vi "Camera Begin.vi"() -> ()   [LabVIEW 2013]
uses:
  <vilib>/Rock Robotics/WPI/Camera/WPI_CameraWhite Balance Values.ctl
  <vilib>/Rock Robotics/WPI/Camera/WPI_CameraFrameRate.ctl
  <vilib>/Rock Robotics/WPI/Camera/WPI_CameraExposure Values.ctl
  <vilib>/Rock Robotics/WPI/Camera/WPI_CameraImageSize.ctl
  <vilib>/Rock Robotics/SystemInterfaces/Typedef/FPGA_TypedefDigitalModule.ctl
  <vilib>/Rock Robotics/SystemInterfaces/DIO/FPGA_DIOPWMChannel.ctl
panel:
  in  "Camera 2":T5={"Camera Address"="192.168.0.90", "Compression"=0, "White Balance"=enum."Auto", "Frame Rate (fps)"=30, "Exposure"=enum."Auto", "Image Size"=enum."320x240", "Brightness"=50, "refnum name"="My Camera RefNum"} {"Brightness" min=0 max=100; "Frame Rate (fps)" min=1 max=30; "Compression" min=0 max=100}
  in  "Camera 1":T5={"Camera Address"="192.168.0.90", "Compression"=0, "White Balance"=enum."Auto", "Frame Rate (fps)"=30, "Exposure"=enum."Auto", "Image Size"=enum."320x240", "Brightness"=50, "refnum name"="My Camera RefNum"} {"Brightness" min=0 max=100; "Frame Rate (fps)" min=1 max=30; "Compression" min=0 max=100}
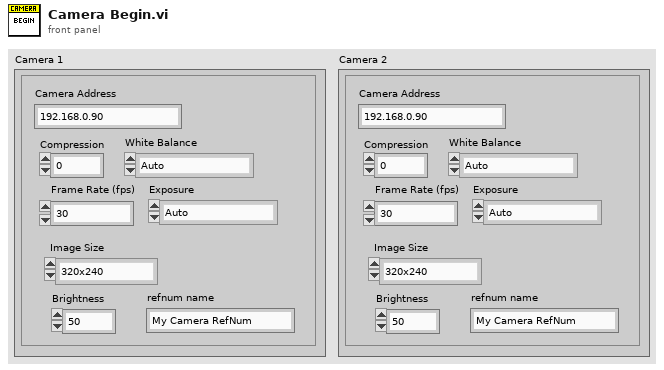
[diagram p1: front panel]
types:
  T1 = typedef "WPI_CameraWhite Balance Values.ctl" = enum16{"Auto", "Fixed indoor", "Fixed outdoor 1", "Fixed outdoor 2", "Fixed fluorescent 1", "Fixed fluorescent 2", "Hold current"}
  T2 = typedef "WPI_CameraFrameRate.ctl" = u32
  T3 = typedef "WPI_CameraExposure Values.ctl" = enum16{"Auto", "Flicker-free 50 Hz", "Flicker-free 60 Hz", "Hold current"}
  T4 = typedef "WPI_CameraImageSize.ctl" = enum16{"640x480", "320x240", "160x120"}
  T5 = cluster{"Camera Address":string, "Compression":i32, "White Balance":T1, "Frame Rate (fps)":T2, "Exposure":T3, "Image Size":T4, "Brightness":i32, "refnum name":string}
  T6 = typedef "FPGA_DIOPWMChannel.ctl" = enum8{"PWM 1", "PWM 2", "PWM 3", "PWM 4", "PWM 5", "PWM 6", "PWM 7", "PWM 8", "PWM 9", "PWM 10", "Invalid"}
  T7 = typedef "FPGA_TypedefDigitalModule.ctl" = enum16{"Digital Module 1", "Digital Module 2"}
  T8 = typedef "WPI_ServoDeviceRef.ctl" = cluster{"DeviceStatus":errorcluster, "Digital Module":T7, "PWM Channel":T6, "DeadBand":T9}
  T9 = typedef "WPI_PWMDeadband.ctl" = cluster{"Name":string, "maxPositivePwm":i32, "minPositivePwm":i32, "centerPwm":i32, "maxNegativePwm":i32, "minNegativePwm":i32, "angularRange":u16}
  T10 = typedef "WPI_CameraDevRef.ctl" = cluster{"Camera Address":string, "CameraStatus":errorcluster, "Acquire Image Notifier":refnum<notifier>}
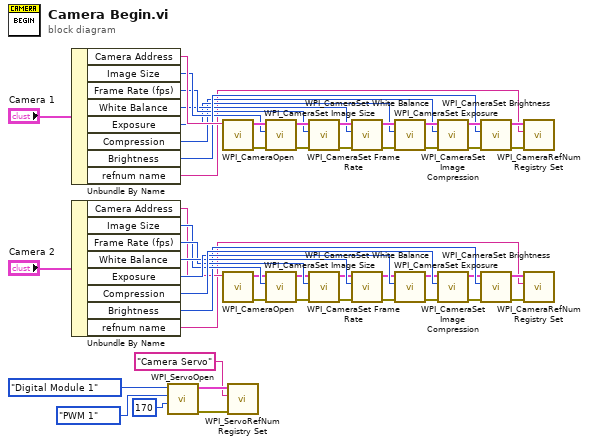
[diagram p0: block diagram]
diagram:
  n1 = Unbundle By Name("Camera 1") -> ("Camera Address"=w37:string, "Image Size"=w35:T4, "Frame Rate (fps)"=w34:T2, "White Balance"=w33:T1, "Exposure"=w32:T3, "Compression"=w31:i32, "Brightness"=w36:i32, "refnum name"=w8:string)
  n2 = Unbundle By Name("Camera 2") -> ("Camera Address"=w24:string, "Image Size"=w26:T4, "Frame Rate (fps)"=w27:T2, "White Balance"=w28:T1, "Exposure"=w29:T3, "Compression"=w30:i32, "Brightness"=w25:i32, "refnum name"=w7:string)
  n3 = call <vilib>:"WPI_ServoOpen.vi"("Angular Range"=u16 170, "PWM Channel"=FPGA_DIOPWMChannel."PWM 1", "Digital Module (Module 1)"=FPGA_TypedefDigitalModule."Digital Module 1") -> ("error out"=w6:errorcluster, "ServoDeviceRef"=w5:T8)  [unwired: 7 in]
  n4 = call <vilib>:"WPI_CameraOpen.vi"("Camera Address"=w37) -> ("error out"=w46:errorcluster, "CameraDevRef"=w47:T10)  [unwired: 1 in, 8 out]
  n5 = call <vilib>:"WPI_CameraOpen.vi"("Camera Address"=w24) -> ("error out"=w15:errorcluster, "CameraDevRef"=w14:T10)  [unwired: 1 in, 8 out]
  n6 = call <vilib>:"WPI_ServoRefNum Registry Set.vi"("error in (no error)"=w6, "refnum name"="Camera Servo", "ServoDeviceRef"=w5) -> ()  [unwired: 7 in, 2 out]
  n7 = call <vilib>:"WPI_CameraSet Image Size.vi"("error in (no error)"=w46, "Image Size"=w35, "CameraDevRef"=w47) -> ("error out"=w45:errorcluster, "CameraDevRef Out"=w48:T10)  [unwired: 7 out]
  n8 = call <vilib>:"WPI_CameraSet Image Size.vi"("error in (no error)"=w15, "Image Size"=w26, "CameraDevRef"=w14) -> ("error out"=w16:errorcluster, "CameraDevRef Out"=w13:T10)  [unwired: 7 out]
  n9 = call <vilib>:"WPI_CameraSet Frame Rate.vi"("error in (no error)"=w45, "Frame Rate (fps)"=w34, "CameraDevRef"=w48) -> ("error out"=w44:errorcluster, "CameraDevRef Out"=w50:T10)  [unwired: 7 out]
  n10 = call <vilib>:"WPI_CameraSet Frame Rate.vi"("error in (no error)"=w16, "Frame Rate (fps)"=w27, "CameraDevRef"=w13) -> ("error out"=w17:errorcluster, "CameraDevRef Out"=w11:T10)  [unwired: 7 out]
  n11 = call <vilib>:"WPI_CameraSet White Balance.vi"("error in (no error)"=w44, "White Balance"=w33, "CameraDevRef"=w50) -> ("error out"=w43:errorcluster, "CameraDevRef Out"=w49:T10)  [unwired: 7 out]
  n12 = call <vilib>:"WPI_CameraSet White Balance.vi"("error in (no error)"=w17, "White Balance"=w28, "CameraDevRef"=w11) -> ("error out"=w18:errorcluster, "CameraDevRef Out"=w12:T10)  [unwired: 7 out]
  n13 = call <vilib>:"WPI_CameraSet Exposure.vi"("error in (no error)"=w43, "Exposure"=w32, "CameraDevRef"=w49) -> ("error out"=w42:errorcluster, "CameraDevRef Out"=w52:T10)  [unwired: 7 out]
  n14 = call <vilib>:"WPI_CameraSet Exposure.vi"("error in (no error)"=w18, "Exposure"=w29, "CameraDevRef"=w12) -> ("error out"=w19:errorcluster, "CameraDevRef Out"=w9:T10)  [unwired: 7 out]
  n15 = call <vilib>:"WPI_CameraSet Image Compression.vi"("error in (no error)"=w42, "Compression"=w31, "CameraDevRef"=w52) -> ("error out"=w41:errorcluster, "CameraDevRef Out"=w51:T10)  [unwired: 7 out]
  n16 = call <vilib>:"WPI_CameraSet Image Compression.vi"("error in (no error)"=w19, "Compression"=w30, "CameraDevRef"=w9) -> ("error out"=w20:errorcluster, "CameraDevRef Out"=w10:T10)  [unwired: 7 out]
  n17 = call <vilib>:"WPI_CameraSet Brightness.vi"("error in (no error)"=w41, "Brightness"=w36, "CameraDevRef"=w51) -> ("error out"=w39:errorcluster, "CameraDevRef Out"=w40:T10)  [unwired: 7 out]
  n18 = call <vilib>:"WPI_CameraSet Brightness.vi"("error in (no error)"=w20, "Brightness"=w25, "CameraDevRef"=w10) -> ("error out"=w22:errorcluster, "CameraDevRef Out"=w21:T10)  [unwired: 7 out]
  n19 = call <vilib>:"WPI_CameraRefNum Registry Set.vi"("error in (no error)"=w39, "refnum name"=w8, "CameraDevRef"=w40) -> ()  [unwired: 9 out]
  n20 = call <vilib>:"WPI_CameraRefNum Registry Set.vi"("error in (no error)"=w22, "refnum name"=w7, "CameraDevRef"=w21) -> ()  [unwired: 9 out]
